vi "Control_a_Motor_With_a_Sensor 1.vi"   [LabVIEW 2015, in "Task 2 Labview.lvrbt"]
doc: "This example is for the LEGO MINDSTORMS NXT. The program runs all motors until a touch sensor is pressed, all motors are then stopped using the brake."
uses:
  Task 2 Labview.lvrbt
  <vilib>/NXT/Block Support/NXT_InputPort.ctl
  <vilib>/NXT/Block Support/NXT_OutputPort.ctl
  <vilib>/NXT/NXTIO Xnodes/NXTIONodeSubVIs/NXTMoveMotors.vi
  <vilib>/NXT/Dual Mode Library/Waits/Wait_Closer.vi
  <vilib>/NXT/NXTIO Xnodes/NXTIONodeSubVIs/NXTStopMotors.vi
  <vilib>/NXT/NXTIO Xnodes/AddressXNode/NXTIOAddress.xnode
  <vilib>/NXT/Subs/LVHSConnector.ctl
  <vilib>/NXT/NXTIO Xnodes/NXTIOXNode/NXTIO.xnode
  <vilib>/NXT/LegoClasses/BrickReference/BrickReference.lvclass
panel:
  # "Control a Motor With a Sensor"
  # "DESCRIPTION\n\nThis program runs all motors until the touch sensor is pressed, then all motors are stopped using the brake.\n\nPORTS \n\nPort A: motor\nPort 1: touch sensor\n\nTIPS \n\n- CTRL-E (PC) or Command-E (Mac) to open the block diagram. \n- This program executes in direct and remote mode."
types:
  T1 = typedef "NXT_InputPort.ctl" = u32
  T2 = typedef "NXT_OutputPort.ctl" = u8
  T3 = typedef "LVHSConnector.ctl" = refnum<class "BrickReference.lvclass">
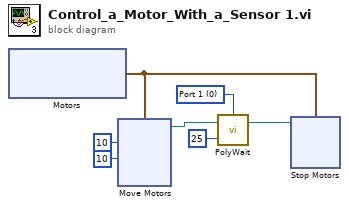
[diagram p0: block diagram]
diagram:
  w7 = T1 0 items=["Port 1", "Port 2", "Port 3", "Port 4"] ("Port (Port 1)")
  n1 = xnode "Motors"() -> ("Motor"=w2:cluster{"Port":T2, "Port":T2})
  n2 = xnode "Move Motors"("Power/Speed 2"=i8 10, "Power/Speed 1"=i8 10, "Motors"=w2) -> ("NXT/EV3"=w4:T3)  [unwired: 1 in]
  n3 = call-poly <vilib>:"PolyWait.vi"("Distance (40)"=i16 25, "NXT/EV3"=w4, "Port (Port 4)"=w7) -> ("NXT/EV3"=w6:T3)  [unwired: 1 in]
  n4 = xnode "Stop Motors"("Motors"=w2, "NXT/EV3"=w6) -> ()  [unwired: 1 out]
